vi "Estrazione Fondo.vi"() -> ()   [LabVIEW 2014]
uses:
  <vilib>/Platform/TimedLoop/XDataNode/timing_clust.ctl
  <vilib>/Platform/TimedLoop/XDataNode/nitl_modes.ctl
  <vilib>/Platform/TimedLoop/XDataNode/wakeup.ctl
  <vilib>/rvi/Emulation/niFpgaGetClockAttributes.vi
  <vilib>/rvi/Emulation/niFpgaSctlEmulationGetInTimedLoop.vi
  <vilib>/rvi/Emulation/niFpgaEmulationReportErrorSimple.vi
  <vilib>/rvi/Emulation/niFpgaCriticalErrorInLSC.vi
  <vilib>/rvi/Emulation/niFpgaEmulationIsFPGAContextNoSignature.vi
  <vilib>/rvi/errors/niFpgaSetErrorForExecOnDevCompSimple.vi
  <vilib>/rvi/eio/common/nirviEmuReportErrorAndStop.vi
  <vilib>/rvi/DataTransferAndStorage/Container/Common/niFpgaContainerGetUniqueNameForEmu.vi
  <vilib>/rvi/FIFO/Fifo_Resource/nirvififoEmulationSetSize.vi
  <vilib>/rvi/FIFO/Fifo_Resource/nirviFifoEmulationQueueMgr.vi
  <instcachedir>/0/nirviFifoEmulationQueueMgr_E5CAEC123FF24DC58D834DCA3CDAA9B5.lvgen/nirviFifoEmulationQueueMgr_E5CAEC123FF24DC58D834DCA3CDAA9B5_010.vi
  <vilib>/rvi/FIFO/Fifo_Resource/nirvififoEmulationCreateLock.vi
  <vilib>/rvi/Emulation/niFpgaProcessEmulError.vi
  <vilib>/rvi/FIFO/Fifo_Resource/nirvififoEmulationObtainLock.vi
  <vilib>/rvi/FIFO/Fifo_Resource/nirvififoEmulationReleaseLock.vi
  <vilib>/rvi/occurrence/nirviWaitOnOccurrenceBase.vi
  <vilib>/rvi/errors/nirviReportUnexpectedCaseInternalError.vi
  <vilib>/rvi/errors/nirviReportUnexpectedCaseInternalError (U32).vi
  <vilib>/rvi/Memory/Memory_Emulation/nirvimemoryFastEmulation.vi
  <vilib>/rvi/Memory/Memory_Emulation/nirvimemoryEmulation.vi
  <vilib>/rvi/FIFO/Fifo_Resource/nirvififoEmulationDetermineInputValidOut.vi
  <vilib>/rvi/eio/common/nirviEmuTemplateMethod_errors.vi
  <vilib>/rvi/interface/RandomDataEmulation/niFpgaRandomDataHandleErrors.vi
  <vilib>/Platform/TimedLoop/XDataNode/XDataNode.xnode
  <vilib>/rvi/DataTransferAndStorage/Container/XNode/niFpgaContainer.xnode
  <vilib>/rvi/FIFO/Fifo_Resource/nirvififoEmulationRead.vi
  <vilib>/rvi/FIFO/Fifo_Resource/nirvififoEmulationWrite.vi
  <vilib>/eio/EIOMethodNode/EIOMethodNode.xnode
  <vilib>/rvi/interface/RandomDataEmulation/nirviRandomDataFpgaReadWriteTemplate.vi
  <vilib>/Platform/TimedLoop/XDataNode/XDNodeRunTimeDep.lvlib
panel:
  in  "N-Mean":i32=8
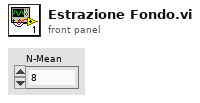
[diagram p1: front panel]
types:
  T1 = typedef "XDNodeRunTimeDep.lvlib/timing_clust.ctl" = cluster{"Expected End [f-1]":u64, "Actual End [f-1]":u64, "Finished Late? [f-1]":bool, "Expected End [i-1]":u64, "Actual End [i-1]":u64, "Finished Late? [i-1]":bool, "Expected Start [i]":u64, "Actual Start [i]":u64, "Expected Start [f]":u64, "Actual Start [f]":u64, "Source Name":string, "Structure Name":string, "Period":i64, "Deadline":i64, "Offset":i64, "Start":i64, "Priority":i32, "Timeout":i32, "Mode":T2, "Wakeup Reason":T3, "Error":errorcluster, "Source Type":string, "Secondary Source Type":string, "Global End Time":u64, "Global Start Time":u64, "Frame Duration":u64, "Iteration Duration":u64, "Assigned CPU":i32, "I/O Scan Engine Mode":u32}
  T2 = typedef "XDNodeRunTimeDep.lvlib/nitl_modes.ctl" = enum32{"No Change", "Process missed periods, maintain original phase", "Discard missed periods, maintain original phase", "Process missed periods, ignore original phase", "Discard missed periods, ignore original phase"}
  T3 = typedef "XDNodeRunTimeDep.lvlib/wakeup.ctl" = enum32{"Normal", "Aborted", "Asynchronous wakeup", "Timing source error", "Timed loop error", "Timeout"}
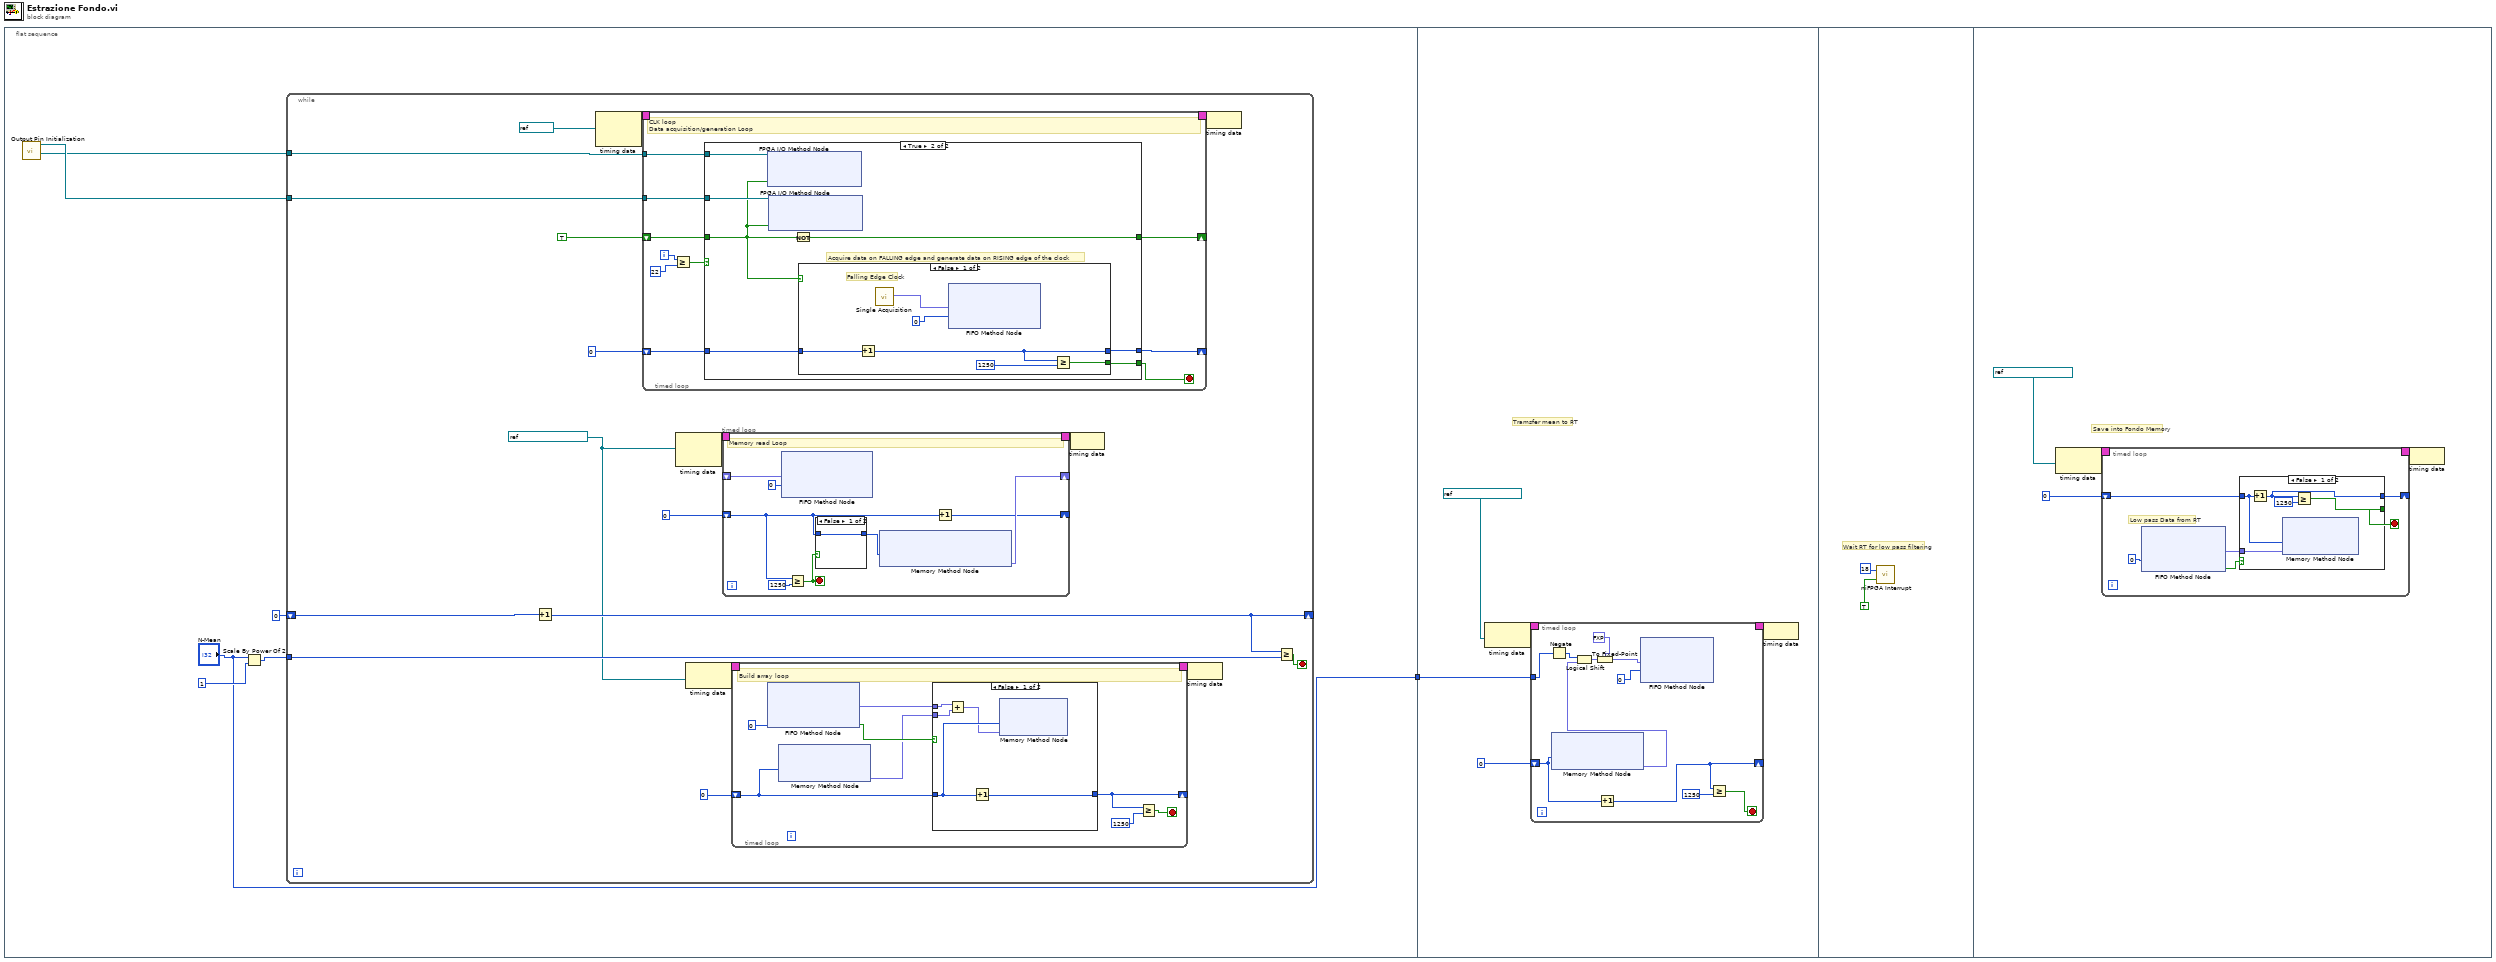
[diagram p0: block diagram]
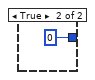
[diagram p2: hidden frame]
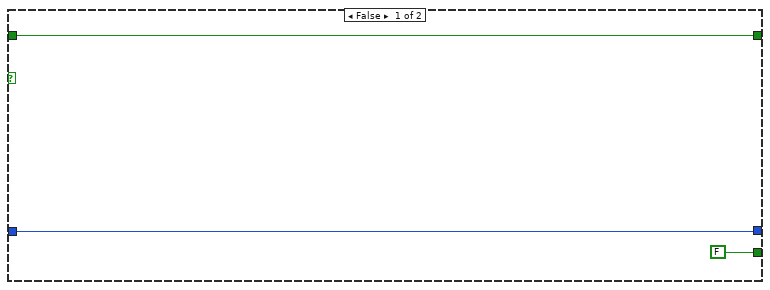
[diagram p4: hidden frame]
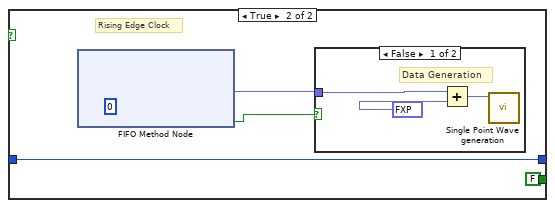
[diagram p5: hidden frame]
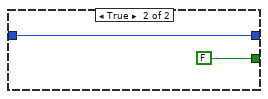
[diagram p7: hidden frame]
diagram:
  n1 = flat-sequence {
    tunnel: ["N-Mean"] -> w1
    tunnel: w1 -> [w102]
    frame #0 {
      n2 = call "Output Pin Initialization.vi"() -> ("I/O Out Clock DAC (pin16)"=w6:refnum<k21>, "I/O Out Clock ADC (pin17)"=w7:refnum<k21>)  [unwired: 8 in, 1 out]
      n3 = Scale By Power Of 2(n="N-Mean", x=1) -> (x*2^n=w3:i32)
      n4 = while {
        shift-right: [w23] -> _
        shift-left: 0 -> [w24]
        tunnel: w7 -> [w20]
        tunnel: w6 -> [w19]
        tunnel: w3 -> [w10]
        stop <- w25 stop-if-true
        w8 = refnum<k21> "40 MHz Onboard Clock" ("Source Name")
        n5 = Increment(x=w24) -> (x+1=w23:i32)
        n6 = node-c288(refnum<k21> "80MHz" ("Source Name")) -> (w22:T1)  [unwired: 1 in]
        n7 = timed-loop {
          timing: w22 -> [_]
          timing-out: [_] -> w21
          shift-right: [w70] -> _
          shift-left: TRUE -> [w68]
          tunnel: w19 -> [w71]
          tunnel: w20 -> [w69]
          shift-right: [w66] -> _
          shift-left: 0 -> [w67]
          i -> [w65]
          stop <- w62 stop-if-true
          # "CLK loop\nData acquisition/generation Loop"
          n8 = Greater Or Equal?(x=w65, y=22) -> (x >= y?=w64:bool)
          n9 = case shown="True" w64 {
            tunnel: w71 -> [_ w81]
            tunnel: [w73 w80] -> w70
            tunnel: w69 -> [_ w79]
            tunnel: w68 -> [w73 w75]
            tunnel: w67 -> [w74 w78]
            tunnel: [FALSE w77] -> w62
            tunnel: [w74 w76] -> w66
            frame False {
            }
            frame True {
              # "Acquire data on FALLING edge and generate data on RISING edge of the clock"
              n10 = xnode "FPGA I/O Method Node"("FPGA I/O In"=w81, "Data"=w75) -> ()  [unwired: 1 out]
              n11 = xnode "FPGA I/O Method Node"("FPGA I/O In"=w79, "Data"=w75) -> ()  [unwired: 1 out]
              n12 = Not(x=w75) -> (.not. x?=w80:bool)
              n13 = case shown="False" w75 {
                tunnel: w78 -> [w87 w89]
                tunnel: [w85 FALSE] -> w77
                tunnel: [w82 w89] -> w76
                frame False {
                  # "Falling Edge Clock"
                  n14 = Increment(x=w87) -> (x+1=w82:i32)
                  n15 = call "Single Acquisition.vi"() -> ("Out"=w84:fxp<+/-,12,12>)  [unwired: 10 in, 1 out]
                  n16 = xnode ("FIFO Method Node")("Element"=w84, "Timeout"=0) -> ()  [unwired: 1 in, 2 out]
                  n17 = Greater Or Equal?(x=w82, y=1250) -> (x >= y?=w85:bool)
                }
                frame True {
                  # "Rising Edge Clock"
                  n18 = xnode ("FIFO Method Node")("Timeout"=0) -> ("Element"=w90:fxp<+/-,12,12>, "Timed Out?"=w91:bool)  [unwired: 1 in, 1 out]
                  n19 = case shown="False" w91 {
                    tunnel: w90 -> [w95 _]
                    frame False {
                      # "Data Generation"
                      n20 = Add(x=w95, y=fxp<+,12,12> 2048.0) -> (x+y=w93:fxp<+/-,14,14>)
                      n21 = call "Single Point Wave generation.vi"("Data To Write"=w93) -> ()  [unwired: 10 in, 1 out]
                    }
                    frame True {
                      # "FPGA memory slow"
                    }
                  }
                }
              }
            }
          }
        }
        n22 = node-c288(w8) -> (w13:T1)  [unwired: 1 in]
        n23 = node-c288(w8) -> (w16:T1)
        n24 = timed-loop {
          timing: w13 -> [_]
          timing-out: [_] -> w12
          shift-right: [w29] -> _
          shift-left: u32 0 -> [w27]
          shift-right: [w31] -> _
          shift-left: _ -> [w30]
          stop <- w28 stop-if-true
          # "Memory read Loop"
          n25 = xnode ("FIFO Method Node")("Element"=w30, "Timeout"=0) -> ()  [unwired: 1 in, 2 out]
          n26 = Greater Or Equal?(x=w27, y=u32 1250) -> (x >= y?=w28:bool)
          n27 = case shown="False" w28 {
            tunnel: w27 -> [w34 _]
            tunnel: [w34 u32 0] -> w26
            frame False {
            }
            frame True {
            }
          }
          n28 = xnode ("Memory Method Node")("Address"=w26) -> ("Data"=w31:fxp<+/-,12,12>)  [unwired: 1 in, 1 out]
          n29 = Increment(x=w27) -> (x+1=w29:u32)
        }
        n30 = timed-loop {
          timing: w16 -> [_]
          timing-out: [_] -> w15
          shift-right: [w47] -> _
          shift-left: u32 0 ("Address") -> [w43]
          stop <- w45 stop-if-true
          # "Build array loop"
          n31 = xnode ("FIFO Method Node")("Timeout"=0) -> ("Element"=w48:fxp<+/-,12,12>, "Timed Out?"=w46:bool)  [unwired: 1 in, 1 out]
          n32 = xnode ("Memory Method Node")("Address"=w43) -> ("Data"=w44:fxp<+/-,24,24>)  [unwired: 1 in, 1 out]
          n33 = case shown="False" w46 {
            tunnel: w48 -> [w52 _]
            tunnel: w43 -> [w53 w55]
            tunnel: [w54 w55] -> w47
            tunnel: w44 -> [w51 _]
            frame False {
              n34 = Add(x=w52, y=w51) -> (x+y=w50:fxp<+/-,24,24>)
              n35 = Increment(x=w53) -> (x+1=w54:u32)
              n36 = xnode ("Memory Method Node")("Address"=w53, "Data"=w50) -> ()  [unwired: 1 in, 1 out]
            }
            frame True {
            }
          }
          n37 = Greater Or Equal?(x=w47, y=u32 1250) -> (x >= y?=w45:bool)
        }
        n38 = node-c288(w12) -> ()
        n39 = node-c288(w15) -> ()
        n40 = node-c288(w21) -> ()
        n41 = Greater Or Equal?(x=w23, y=w10) -> (x >= y?=w25:bool)
      }
    }
    frame #1 {
      # "Tramsfer mean to RT"
      n42 = node-c288(refnum<k21> "40 MHz Onboard Clock" ("Source Name")) -> (w106:T1)
      n43 = timed-loop {
        tunnel: w102 -> [w108]
        timing: w106 -> [_]
        timing-out: [_] -> w105
        shift-right: [w115] -> _
        shift-left: u32 0 ("Address") -> [w116]
        stop <- w114 stop-if-true
        n44 = Negate(x=w108) -> (-x=w107:i32)
        n45 = xnode ("Memory Method Node")("Address"=w116) -> ("Data"=w112:fxp<+/-,24,24>)  [unwired: 1 in, 1 out]
        n46 = Logical Shift(y=w107, x=w112) -> (x << y=w111:fxp<+/-,24,24>)
        n47 = To Fixed-Point(fixed-point type=fxp<+/-,12,12> 0.0 ("Element"), number=w111) -> (fixed-point=w110:fxp<+/-,12,12>)
        n48 = Increment(x=w116) -> (x+1=w115:u32)
        n49 = xnode ("FIFO Method Node")("Element"=w110, "Timeout"=0) -> ()  [unwired: 1 in, 2 out]
        n50 = Greater Or Equal?(x=w115, y=u32 1250) -> (x >= y?=w114:bool)
      }
      n51 = node-c288(w105) -> ()
    }
    frame #2 {
      # "Wait RT for low pass filtering"
      n52 = call <vilib>:"niFPGA Interrupt.vi"("Wait Until Cleared (F)"=TRUE, "IRQ Number (0)"=u8 18) -> ()  [unwired: 1 in]
    }
    frame #3 {
      # "Save into Fondo Memory"
      n53 = node-c288(refnum<k21> "40 MHz Onboard Clock" ("Source Name")) -> (w129:T1)
      n54 = timed-loop {
        timing: w129 -> [_]
        timing-out: [_] -> w128
        shift-right: [w131] -> _
        shift-left: u32 0 ("Address") -> [w133]
        stop <- w132 stop-if-true
        # "Low pass Data from RT"
        n55 = xnode ("FIFO Method Node")("Timeout"=0) -> ("Element"=w134:fxp<+/-,12,12>, "Timed Out?"=w130:bool)  [unwired: 1 in, 1 out]
        n56 = case shown="False" w130 {
          tunnel: w134 -> [w140 _]
          tunnel: w133 -> [w139 w142]
          tunnel: [w138 FALSE] -> w132
          tunnel: [w137 w142] -> w131
          frame False {
            n57 = Increment(x=w139) -> (x+1=w137:u32)
            n58 = xnode ("Memory Method Node")("Address"=w139, "Data"=w140) -> ()  [unwired: 1 in, 1 out]
            n59 = Greater Or Equal?(x=w137, y=u32 1250) -> (x >= y?=w138:bool)
          }
          frame True {
          }
        }
      }
      n60 = node-c288(w128) -> ()
    }
  }
